vi "appendXMLYCalibration.vi"(3 "error in (no error)":errorcluster, 4 "YCalibration":cluster{dbl, dbl}[](graph), 5 "Parent Device Node":refnum<k20>, 6 "DOM document in":refnum<k20>) -> (0 "error out":errorcluster)   [LabVIEW 2013]
uses:
  <resource>/objmgr/DOMUserDefRef.rc
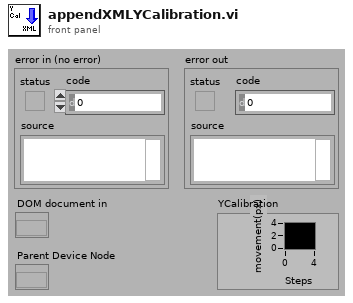
[diagram p1: front panel]
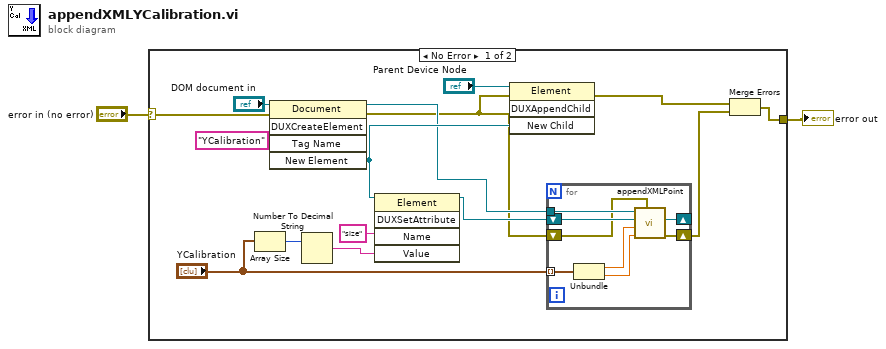
[diagram p0: block diagram]
diagram:
  n1 = case shown="No Error" "error in (no error)" {
    selector: "error in (no error)" -> [w14 w26]
    tunnel: [w3 w26] -> w2
    frame No Error {
      n2 = Array Size(array="YCalibration") -> (size(s)=w10:i32)
      n3 = invoke class="Document" method="DUXCreateElement"(reference="DOM document in", error in=w14, "Tag Name"="YCalibration") -> (reference out=w7:refnum<k20>, error out=w6:errorcluster, "New Element"=w13:refnum<k20>)  [unwired: 2 in, 2 out]
      n4 = Number To Decimal String(number=w10) -> (decimal integer string=w9:string)  [unwired: 1 in]
      n5 = invoke class="Element" method="DUXSetAttribute"(reference=w13, "Name"="size", "Value"=w9) -> (reference out=w8:refnum<k20>)  [unwired: 2 in, 4 out]
      n6 = invoke class="Element" method="DUXAppendChild"(reference="Parent Device Node", error in=w6, "New Child"=w13) -> (error out=w4:errorcluster)  [unwired: 1 in, 3 out]
      n7 = for {
        tunnel: "YCalibration" -> [w25] mode=indexing
        shift-right: [w22] -> _
        shift-left: w8 -> [w21]
        tunnel: w7 -> [w20]
        shift-right: [w19] -> w5
        shift-left: w6 -> [w18]
        n8 = Unbundle(w25) -> (w24:dbl, w23:dbl)
        n9 = call "appendXMLPoint.vi"("error in (no error)"=w18, "y"=w23, "x"=w24, "Parent Node"=w21, "DOM document in"=w20) -> ("error out"=w19:errorcluster, "Parent Node Out"=w22:refnum<k20>)  [unwired: 4 in]
      }
      n10 = Merge Errors(w4, w5) -> (w3:errorcluster)
    }
    frame Error {
    }
  }
  "error out" <- w2
